vi "卡件上位机界面.vi"() -> ()   [LabVIEW 2013]
panel:
  in  "Tab Control":enum32{"Page 1", "Page 2"}(tab)
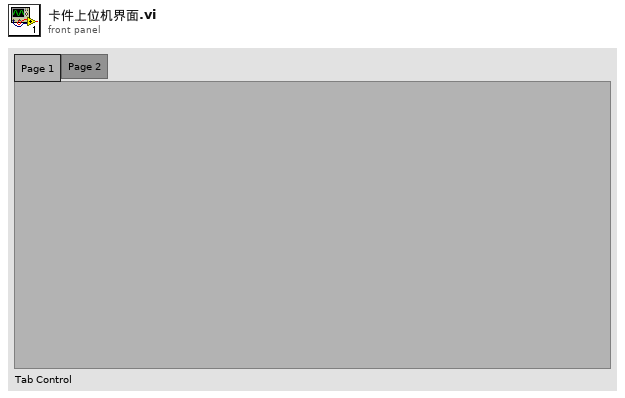
[diagram p1: front panel]
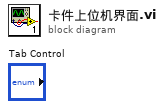
[diagram p0: block diagram]
diagram:
